vi "UTIL Initialize Moving Average.vi"(8 "Error In":errorcluster, 11 "Window Width":i32=20) -> (0 "Error Out":errorcluster, 3 "queue out":refnum<queue>)   [LabVIEW 2017]
doc: "Initialize a Moving Window Average routine by creating a fixed-length, Windows-sized Queue of Dbls, and initializing them to 0.\n\nInput:\n Window Size I32, default 10\n Error In\nOutput:\n Average Queue Fixed-length Queue of Dbl\n Error Out"
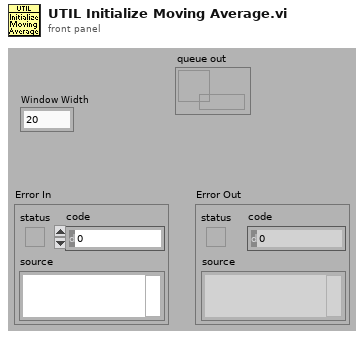
[diagram p1: front panel]
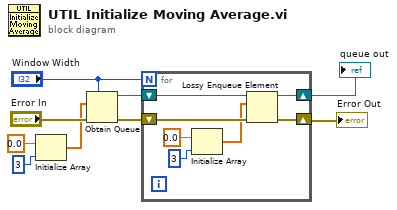
[diagram p0: block diagram]
diagram:
  n1 = Initialize Array(0.0 ("element"), 3 ("dimension size")) -> (w2:dbl[])
  n2 = Obtain Queue(max queue size (-1, unlimited)="Window Width", element data type=w2, error in (no error)="Error In") -> (queue out=w8:refnum<queue>, error out=w9:errorcluster)  [unwired: 2 in, 1 out]
  n3 = for {
    N: "Window Width" -> [_]
    shift-right: [w15] -> w6
    shift-left: w9 -> [w16]
    shift-right: [w13] -> w1
    shift-left: w8 -> [w14]
    n4 = Initialize Array(0.0 ("element"), 3 ("dimension size")) -> (w10:dbl[])
    n5 = Lossy Enqueue Element(queue=w14, element=w10, error in (no error)=w16) -> (queue out=w13:refnum<queue>, error out=w15:errorcluster)  [unwired: 2 out]
  }
  "Error Out" <- w6
  "queue out" <- w1
